vi "StimulationMode.vi"(8 "error in (no error)":errorcluster, 11 "SetupInfo_IN":T1={"ConfigParameters_Analog"={"JAI camera fps"=240.0, "Bi-Lateral Galvo xy scan range (V)"=0.7, "Bi-Lateral Galvo xy scan frequency (Hz)"=500, "AOM Blind percent (%)"=0.1, "AOM start blind percent (%) "=70.0, "ROI threshold"=1.0, "AO Sampling rate"=1000000.0}, "ConfigParameters_Digital"={"Steps per volume"=25.0, "Time per volume (s)"=0.4, "OG start layer"=15.0, "Objective Lin Rising Vel (micron/ms）"=1.0, "Image depth (micron)"=200.0, "OG latency (s)"=10.0, "OG repitation"=3.0, "OG end layer"=17.0, "Shock1 duration (s)"=0.001, "Shock2 duration (s)"=0.001, "Shock3 duration (s)"=0.01, "Shock4 duration (s)"=0.01, "Shock5 duration (s)"=0.1, "Shock duration_New"=[]}, "ConfigParameters_Other1"={"Frontal Galvo xy scan range (V)"=0.14, "Frontal Galvo xy scan frequency (Hz)"=500, "PFI 0 digital clock frequency"=500000.0, "Window size for layer index"=0.5, "sCMOS fps"=95.0}, "ConfigParameters_Others2"={"#Trials baseline"=6, "#Trials test"=6, "Time before acq. (s)"=360.0, "Time before test (s)"=600.0, "#Blocks acquisition"=5, "Inter-trial interval baseline (s)"=60.0, "#Trials per acquition block"=6, "Inter-block interval acquisition (s)"=360.0, "Inter-trial interval acquisition (s)"=20.0, "Flash latency (s)"=10.0, "Flash duration (s)"=3.2, "Response duration (s)"=10.0, "MaxTimeEventDetection (s)"=6, "StimType"=enum."Flash", "#MaxEvents"=6}, "ProcessParametersOut"={"stand Z vol Acquisition time (s)"=0.2631578947368421, "stand Z vol Backward time (s)"=0.13684210526315793, "Objective scan volt"=5.0, "Bi-lateral Galvo Z scan volt"=0.1800000180000018, "Frontal Galvo Z scan volt"=0.14940000509752818, "Objective step length (micron)"=8.0, "OG Z volet Linear Dec time (s)"=0.024, "OG Z vol Stim. steps time (s)"=0.031578947368421054, "OG Z vol Linear Acc time (s)"=0.112, "#Vol. of flash"=8, "#Vol. of shock"=1, "#Vol. bef flash"=25, "#Vol. aft flash"=17, "OG Z vol Linear Dec time (s)"=0.112, "OG Z vol time (s)"=0.39073684210526316, "Stack duration"=[0.001, 0.001, 0.01, 0.01, 0.1], "AOM stand. value size"=400000, "Plane indexing length"=0, "#Vol. blank"=0, "#Vol. blank before acq"=1000000, "#Vol. blank before test"=263158, " #Inter-block interval acquisition (Ed-St Vol)"=1000000}, "WaveformParameters"={"stand Z vol Acquisition samp info"={"Fs"=1000000.0, "#s"=263158.0}, "stand Z vol Backward samp info"={"Fs"=1000000.0, "#s"=136842.0}, "OG Z vol Linear Acc samp info"={"Fs"=1000000.0, "#s"=112000.0}, "OG Z vol Stim. steps samp info"={"Fs"=1000000.0, "#s"=31579.0}, "OG Z volet Linear Dec samp info"={"Fs"=1000000.0, "#s"=24000.0}, "OG Z vol Linear Dec samp info"={"Fs"=1000000.0, "#s"=112000.0}, "OG Z vol samp info"={"Fs"=1000000.0, "#s"=390737.0}, "stand Z vol backforth samp info"={"Fs"=1000000.0, "#s"=400000.0}}, "AnalogWaveform"={"Bi-lateral Galvo Z stand waveform"={"t0"=timestamp(0 s since 1904-01-01), "dt"=1.0, "Y"=[]}, "Frontal Galvo Z stand waveform"={"t0"=timestamp(0 s since 1904-01-01), "dt"=1.0, "Y"=[]}, "Bi-lateral Galvo XY stand waveform"={"t0"=timestamp(0 s since 1904-01-01), "dt"=1.0, "Y"=[]}, "Frontal Galvo XY stand waveform"={"t0"=timestamp(0 s since 1904-01-01), "dt"=1.0, "Y"=[]}, "sCMOS stand waveform"={"t0"=timestamp(0 s since 1904-01-01), "dt"=1.0, "Y"=[]}, "Detection objective stand waveform"={"t0"=timestamp(0 s since 1904-01-01), "dt"=1.0, "Y"=[]}, "AOM stand waveform"={"t0"=timestamp(0 s since 1904-01-01), "dt"=1.0, "Y"=[]}, "PFI 0 clock stand waveform"={"t0"=timestamp(0 s since 1904-01-01), "dt"=1.0, "Y"=[]}, "Bi-lateral Galvo Z OG waveform"={"t0"=timestamp(0 s since 1904-01-01), "dt"=1.0, "Y"=[]}, "Bi-lateral Galvo XY OG waveform"={"t0"=timestamp(0 s since 1904-01-01), "dt"=1.0, "Y"=[]}, "Frontal Galvo Z OG waveform"={"t0"=timestamp(0 s since 1904-01-01), "dt"=1.0, "Y"=[]}, "Frontal Galvo XY OG waveform"={"t0"=timestamp(0 s since 1904-01-01), "dt"=1.0, "Y"=[]}, "sCMOS OG waveform"={"t0"=timestamp(0 s since 1904-01-01), "dt"=1.0, "Y"=[]}, "Detection objective OG waveform"={"t0"=timestamp(0 s since 1904-01-01), "dt"=1.0, "Y"=[]}, "AOM OG waveform"={"t0"=timestamp(0 s since 1904-01-01), "dt"=1.0, "Y"=[]}, "PFI 0 clock OG wavee"={"t0"=timestamp(0 s since 1904-01-01), "dt"=1.0, "Y"=[]}, "sCMOS blank waveform"={"t0"=timestamp(0 s since 1904-01-01), "dt"=1.0, "Y"=[]}, "All analog OG wave"=[], "All analog stand wave"=[], "All analog blank wave"=[], "BufferWaveform_Analog"=[], "Bi-lateral Galvo Z XY"={"t0"=timestamp(0 s since 1904-01-01), "dt"=1.0, "Y"=[]}, "Frontal Galvo Z XY"={"t0"=timestamp(0 s since 1904-01-01), "dt"=1.0, "Y"=[]}, "sCMOS Trigger XY"={"t0"=timestamp(0 s since 1904-01-01), "dt"=1.0, "Y"=[]}, "Detection objective XY"={"t0"=timestamp(0 s since 1904-01-01), "dt"=1.0, "Y"=[]}, "AOM XY"={"t0"=timestamp(0 s since 1904-01-01), "dt"=1.0, "Y"=[]}, "Analog_XY"=[]}, "DigitalWaveform"={"AllDigitalStandWave"=[], "AllDigialEvokedWave"=[], "AllDigialOGWave"=[], "AllDigitalPairWave_1"=[], "AllDigitalPairWave_2"=[], "AllDigitalPairWave_3"=[], "AllDigitalPairWave_4"=[], "AllDigitalPairWave_5"=[], "Plane Indexing"={"t0"=timestamp(0 s since 1904-01-01), "dt"=0.0, "Y"={"transitions"=[], "data"=[]}, "error"={"status"=FALSE, "code"=37421928, "source"=""}}, "Plane indexing P0.5 OG"={"t0"=timestamp(0 s since 1904-01-01), "dt"=0.0, "Y"={"transitions"=[], "data"=[]}, "error"={"status"=FALSE, "code"=37421928, "source"=""}}, "AllDigitalPairWaves"=[], "BufferWaveform_Digital"=[], "AllDigitalBlankWave"=[], "Digial_XY"=[], "Digital_XY_flash"=[], "Digial_XY DMD"=[]}, "PhysicalResource"={"PhysicalChannels_AI"="", "PhysicalChannels_AO"="", "PhysicalChannels_DO"="", "Task_AnalogOutput"="", "Task_DigitalOutput"="", "Task_AnalogInput"=""}, "ControlsRef"={"Mode_1"=refnum, "EventDetectionMode"=refnum, "Mode_2A"=refnum, "StimulationMode"=refnum, "Mode_2B"=refnum, "ErrorMeg"=refnum}, "test"=""} {"ConfigParameters_Other1"."Frontal Galvo xy scan frequency (Hz)" min=500 max=500; "ConfigParameters_Other1"."Frontal Galvo xy scan range (V)" min=0.0 max=1.5; "ConfigParameters_Analog"."AOM start blind percent (%)" min=10.0 max=90.0; "ConfigParameters_Analog"."AOM Blind percent (%)" min=0.1 max=100.0; "ConfigParameters_Analog"."Bi-Lateral Galvo xy scan frequency (Hz)" min=500 max=500; "ConfigParameters_Analog"."Bi-Lateral Galvo xy scan range (V)" min=0.0 max=1.5}) -> (0 "error out":errorcluster, 3 "SetupInfo_OUT":T1={"ConfigParameters_Analog"={"JAI camera fps"=240.0, "Bi-Lateral Galvo xy scan range (V)"=0.7, "Bi-Lateral Galvo xy scan frequency (Hz)"=500, "AOM Blind percent (%)"=0.1, "AOM start blind percent (%) "=70.0, "ROI threshold"=1.0, "AO Sampling rate"=1000000.0}, "ConfigParameters_Digital"={"Steps per volume"=25.0, "Time per volume (s)"=0.4, "OG start layer"=15.0, "Objective Lin Rising Vel (micron/ms）"=1.0, "Image depth (micron)"=200.0, "OG latency (s)"=10.0, "OG repitation"=3.0, "OG end layer"=17.0, "Shock1 duration (s)"=0.001, "Shock2 duration (s)"=0.001, "Shock3 duration (s)"=0.01, "Shock4 duration (s)"=0.01, "Shock5 duration (s)"=0.1, "Shock duration_New"=[]}, "ConfigParameters_Other1"={"Frontal Galvo xy scan range (V)"=0.14, "Frontal Galvo xy scan frequency (Hz)"=500, "PFI 0 digital clock frequency"=500000.0, "Window size for layer index"=0.5, "sCMOS fps"=95.0}, "ConfigParameters_Others2"={"#Trials baseline"=6, "#Trials test"=6, "Time before acq. (s)"=360.0, "Time before test (s)"=600.0, "#Blocks acquisition"=5, "Inter-trial interval baseline (s)"=60.0, "#Trials per acquition block"=6, "Inter-block interval acquisition (s)"=360.0, "Inter-trial interval acquisition (s)"=20.0, "Flash latency (s)"=10.0, "Flash duration (s)"=3.2, "Response duration (s)"=10.0, "MaxTimeEventDetection (s)"=6, "StimType"=enum."Flash", "#MaxEvents"=6}, "ProcessParametersOut"={"stand Z vol Acquisition time (s)"=0.2631578947368421, "stand Z vol Backward time (s)"=0.13684210526315793, "Objective scan volt"=5.0, "Bi-lateral Galvo Z scan volt"=0.1800000180000018, "Frontal Galvo Z scan volt"=0.14940000509752818, "Objective step length (micron)"=8.0, "OG Z volet Linear Dec time (s)"=0.024, "OG Z vol Stim. steps time (s)"=0.031578947368421054, "OG Z vol Linear Acc time (s)"=0.112, "#Vol. of flash"=8, "#Vol. of shock"=1, "#Vol. bef flash"=25, "#Vol. aft flash"=17, "OG Z vol Linear Dec time (s)"=0.112, "OG Z vol time (s)"=0.39073684210526316, "Stack duration"=[0.001, 0.001, 0.01, 0.01, 0.1], "AOM stand. value size"=400000, "Plane indexing length"=0, "#Vol. blank"=0, "#Vol. blank before acq"=1000000, "#Vol. blank before test"=263158, " #Inter-block interval acquisition (Ed-St Vol)"=1000000}, "WaveformParameters"={"stand Z vol Acquisition samp info"={"Fs"=1000000.0, "#s"=263158.0}, "stand Z vol Backward samp info"={"Fs"=1000000.0, "#s"=136842.0}, "OG Z vol Linear Acc samp info"={"Fs"=1000000.0, "#s"=112000.0}, "OG Z vol Stim. steps samp info"={"Fs"=1000000.0, "#s"=31579.0}, "OG Z volet Linear Dec samp info"={"Fs"=1000000.0, "#s"=24000.0}, "OG Z vol Linear Dec samp info"={"Fs"=1000000.0, "#s"=112000.0}, "OG Z vol samp info"={"Fs"=1000000.0, "#s"=390737.0}, "stand Z vol backforth samp info"={"Fs"=1000000.0, "#s"=400000.0}}, "AnalogWaveform"={"Bi-lateral Galvo Z stand waveform"={"t0"=timestamp(0 s since 1904-01-01), "dt"=1.0, "Y"=[]}, "Frontal Galvo Z stand waveform"={"t0"=timestamp(0 s since 1904-01-01), "dt"=1.0, "Y"=[]}, "Bi-lateral Galvo XY stand waveform"={"t0"=timestamp(0 s since 1904-01-01), "dt"=1.0, "Y"=[]}, "Frontal Galvo XY stand waveform"={"t0"=timestamp(0 s since 1904-01-01), "dt"=1.0, "Y"=[]}, "sCMOS stand waveform"={"t0"=timestamp(0 s since 1904-01-01), "dt"=1.0, "Y"=[]}, "Detection objective stand waveform"={"t0"=timestamp(0 s since 1904-01-01), "dt"=1.0, "Y"=[]}, "AOM stand waveform"={"t0"=timestamp(0 s since 1904-01-01), "dt"=1.0, "Y"=[]}, "PFI 0 clock stand waveform"={"t0"=timestamp(0 s since 1904-01-01), "dt"=1.0, "Y"=[]}, "Bi-lateral Galvo Z OG waveform"={"t0"=timestamp(0 s since 1904-01-01), "dt"=1.0, "Y"=[]}, "Bi-lateral Galvo XY OG waveform"={"t0"=timestamp(0 s since 1904-01-01), "dt"=1.0, "Y"=[]}, "Frontal Galvo Z OG waveform"={"t0"=timestamp(0 s since 1904-01-01), "dt"=1.0, "Y"=[]}, "Frontal Galvo XY OG waveform"={"t0"=timestamp(0 s since 1904-01-01), "dt"=1.0, "Y"=[]}, "sCMOS OG waveform"={"t0"=timestamp(0 s since 1904-01-01), "dt"=1.0, "Y"=[]}, "Detection objective OG waveform"={"t0"=timestamp(0 s since 1904-01-01), "dt"=1.0, "Y"=[]}, "AOM OG waveform"={"t0"=timestamp(0 s since 1904-01-01), "dt"=1.0, "Y"=[]}, "PFI 0 clock OG wavee"={"t0"=timestamp(0 s since 1904-01-01), "dt"=1.0, "Y"=[]}, "sCMOS blank waveform"={"t0"=timestamp(0 s since 1904-01-01), "dt"=1.0, "Y"=[]}, "All analog OG wave"=[], "All analog stand wave"=[], "All analog blank wave"=[], "BufferWaveform_Analog"=[], "Bi-lateral Galvo Z XY"={"t0"=timestamp(0 s since 1904-01-01), "dt"=1.0, "Y"=[]}, "Frontal Galvo Z XY"={"t0"=timestamp(0 s since 1904-01-01), "dt"=1.0, "Y"=[]}, "sCMOS Trigger XY"={"t0"=timestamp(0 s since 1904-01-01), "dt"=1.0, "Y"=[]}, "Detection objective XY"={"t0"=timestamp(0 s since 1904-01-01), "dt"=1.0, "Y"=[]}, "AOM XY"={"t0"=timestamp(0 s since 1904-01-01), "dt"=1.0, "Y"=[]}, "Analog_XY"=[]}, "DigitalWaveform"={"AllDigitalStandWave"=[], "AllDigialEvokedWave"=[], "AllDigialOGWave"=[], "AllDigitalPairWave_1"=[], "AllDigitalPairWave_2"=[], "AllDigitalPairWave_3"=[], "AllDigitalPairWave_4"=[], "AllDigitalPairWave_5"=[], "Plane Indexing"={"t0"=timestamp(0 s since 1904-01-01), "dt"=0.0, "Y"={"transitions"=[], "data"=[]}, "error"={"status"=FALSE, "code"=37421928, "source"=""}}, "Plane indexing P0.5 OG"={"t0"=timestamp(0 s since 1904-01-01), "dt"=0.0, "Y"={"transitions"=[], "data"=[]}, "error"={"status"=FALSE, "code"=37421928, "source"=""}}, "AllDigitalPairWaves"=[], "BufferWaveform_Digital"=[], "AllDigitalBlankWave"=[], "Digial_XY"=[], "Digital_XY_flash"=[], "Digial_XY DMD"=[]}, "PhysicalResource"={"PhysicalChannels_AI"="", "PhysicalChannels_AO"="", "PhysicalChannels_DO"="", "Task_AnalogOutput"="", "Task_DigitalOutput"="", "Task_AnalogInput"=""}, "ControlsRef"={"Mode_1"=refnum, "EventDetectionMode"=refnum, "Mode_2A"=refnum, "StimulationMode"=refnum, "Mode_2B"=refnum, "ErrorMeg"=refnum}, "test"=""} {"ConfigParameters_Other1"."Frontal Galvo xy scan frequency (Hz)" min=500 max=500; "ConfigParameters_Other1"."Frontal Galvo xy scan range (V)" min=0.0 max=1.5; "ConfigParameters_Analog"."AOM start blind percent (%)" min=10.0 max=90.0; "ConfigParameters_Analog"."AOM Blind percent (%)" min=0.1 max=100.0; "ConfigParameters_Analog"."Bi-Lateral Galvo xy scan frequency (Hz)" min=500 max=500; "ConfigParameters_Analog"."Bi-Lateral Galvo xy scan range (V)" min=0.0 max=1.5})   [LabVIEW 2018]
uses:
  SetupInfo.ctl
  ConfigParameters_Analog.ctl
  ConfigParameters_Digital.ctl
  ConfigParameters_Others1.ctl
  ConfigParameters_Others2.ctl
  ProcessParametersOut.ctl
  WaveformParameters.ctl
  AnalogWaveform.ctl
  DigitalWaveform.ctl
  PhysicalResource.ctl
  ControlsRef.ctl
  <vilib>/DAQmx/write.llb/DAQmx Write (Analog DBL 1Chan 1Samp).vi
  <vilib>/Analysis/baseanly.llb/Mean (DBL).vi
  <vilib>/DAQmx/create/channels.llb/DAQmx Create Channel (AO-Voltage-Basic).vi
  <vilib>/DAQmx/miscellaneous.llb/DAQmx Fill In Error Info.vi
  Trigger_Global.vi
  <vilib>/Analysis/NI_AALBase.lvlib
panel:
  out "OG?":bool
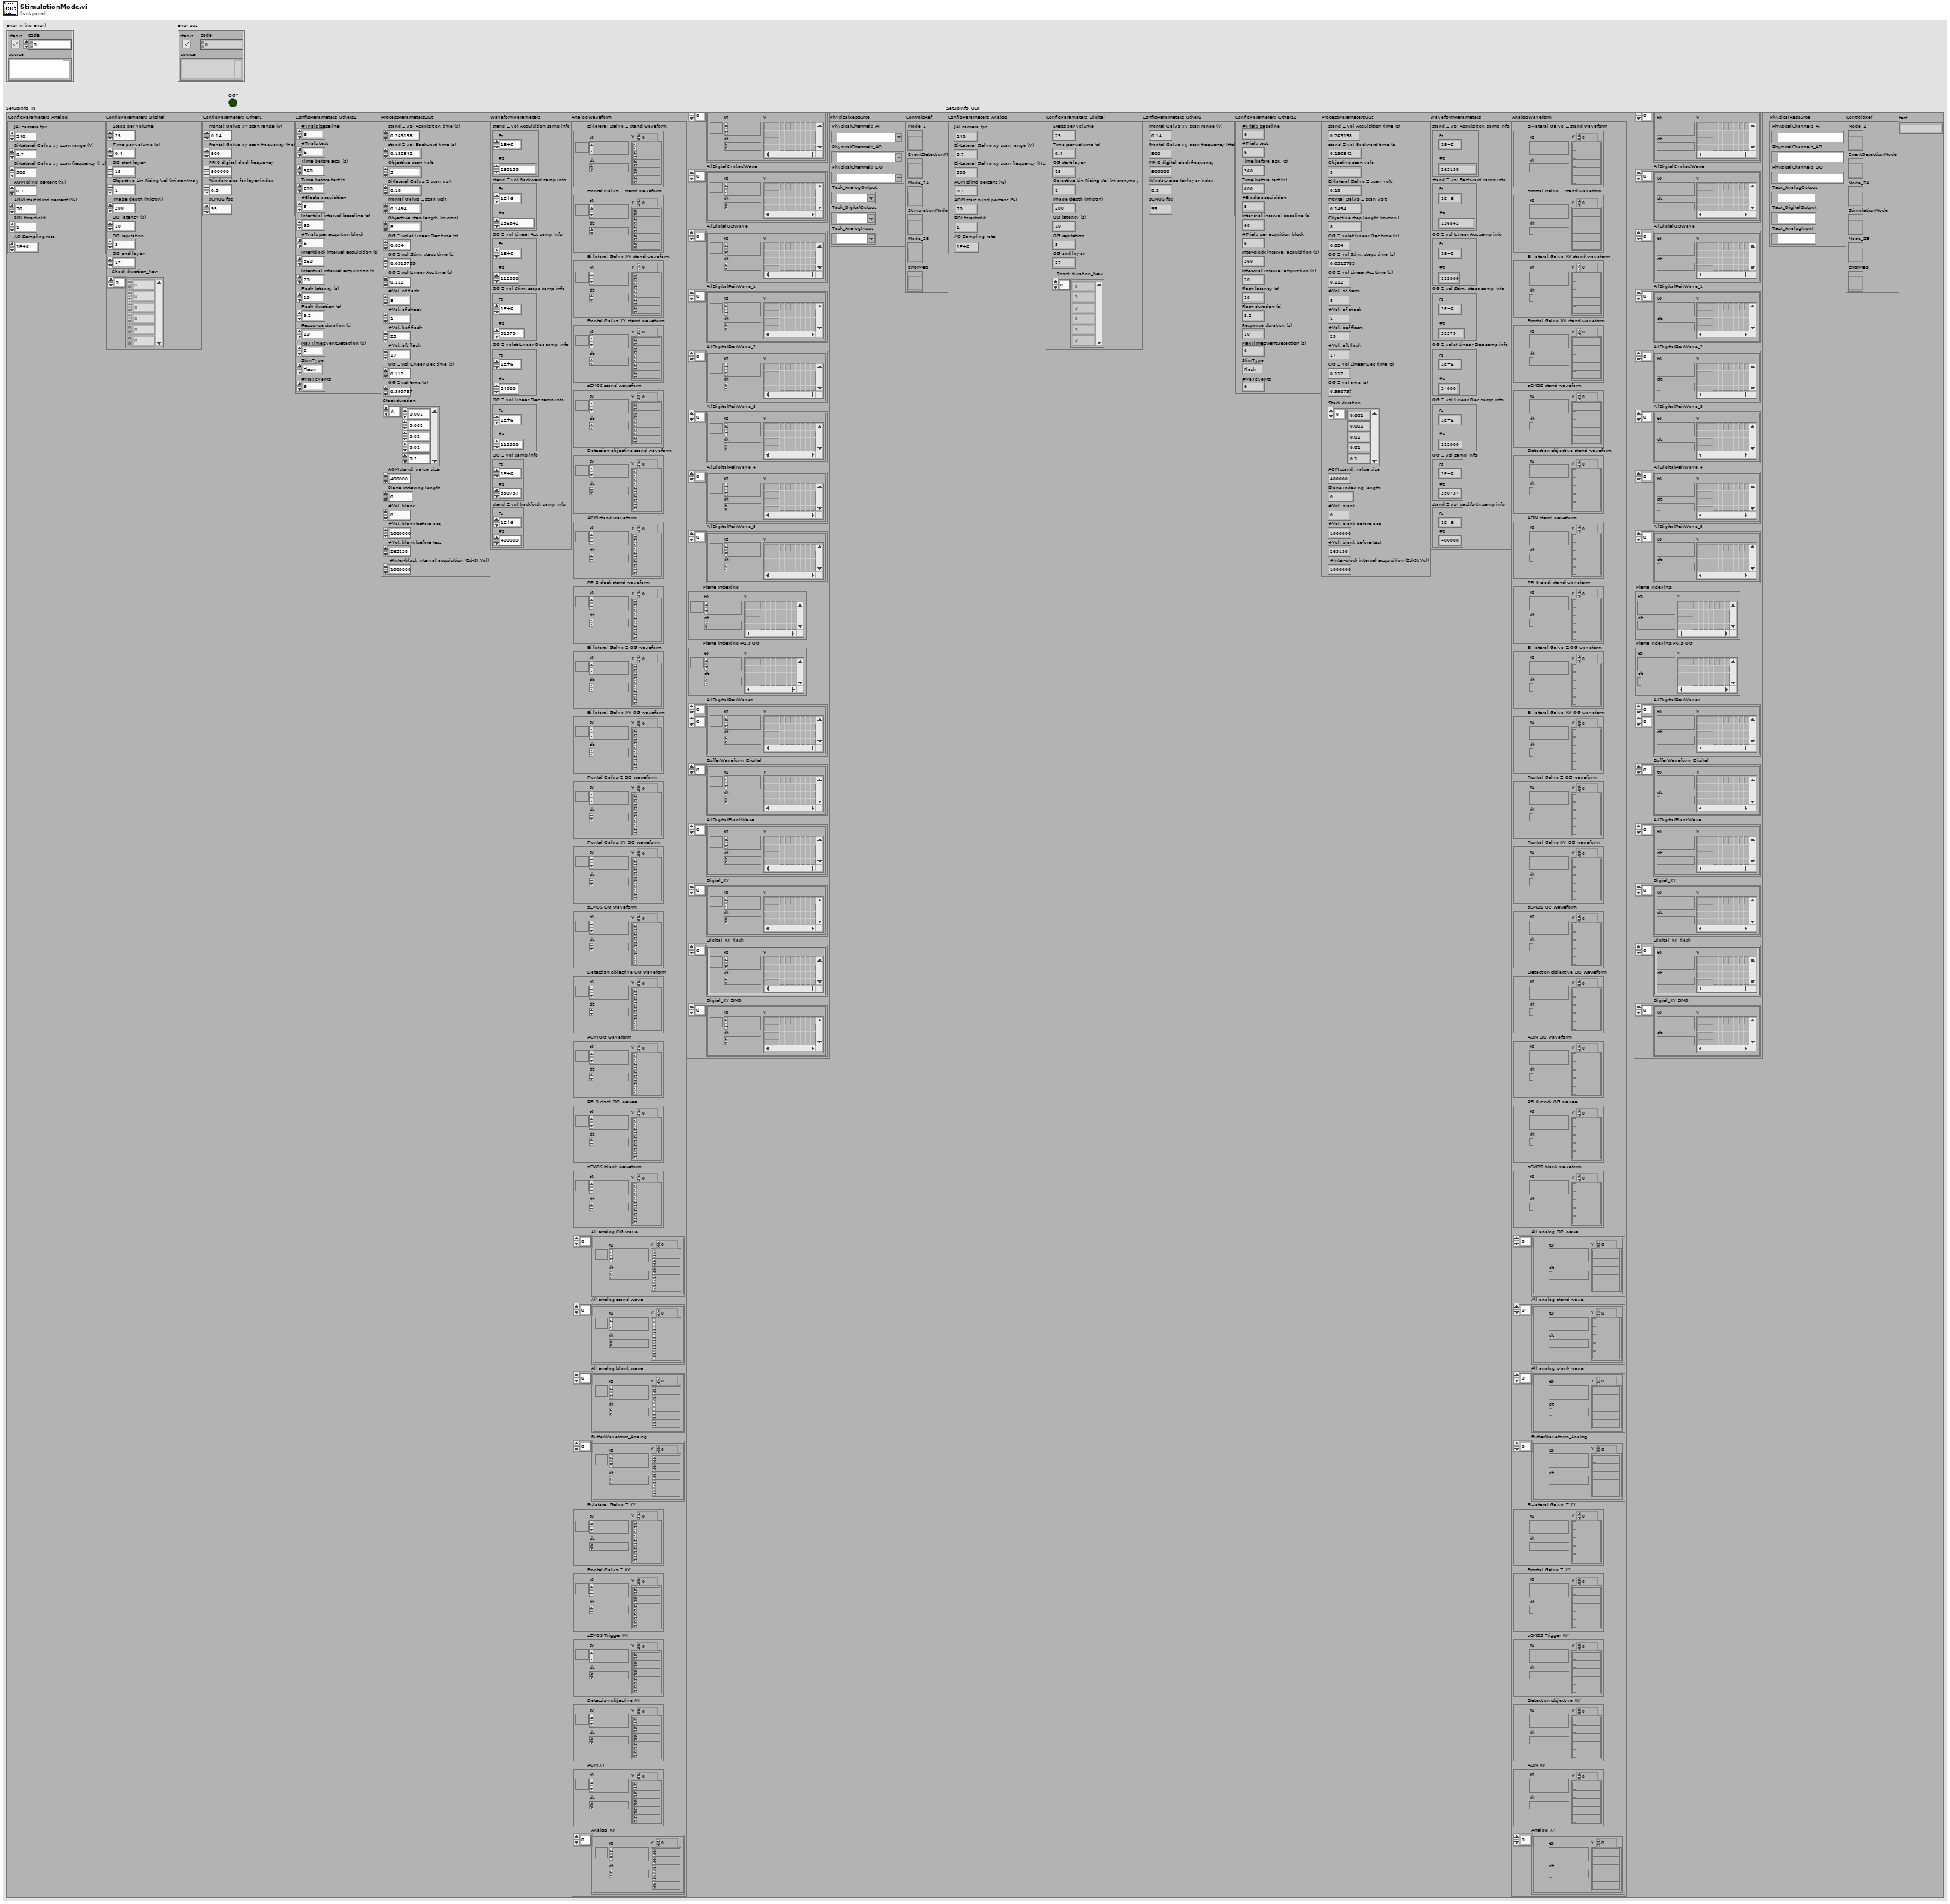
[diagram p1: front panel]
types:
  T1 = typedef "SetupInfo.ctl" = cluster{"ConfigParameters_Analog":T2, "ConfigParameters_Digital":T3, "ConfigParameters_Other1":T4, "ConfigParameters_Others2":T5, "ProcessParametersOut":T6, "WaveformParameters":T7, "AnalogWaveform":T8, "DigitalWaveform":T9, "PhysicalResource":T10, "ControlsRef":T11, "test":string}
  T2 = typedef "ConfigParameters_Analog.ctl" = cluster{"JAI camera fps":dbl, "Bi-Lateral Galvo xy scan range (V)":dbl, "Bi-Lateral Galvo xy scan frequency (Hz)":i16, "AOM Blind percent (%)":dbl, "AOM start blind percent (%) ":dbl, "ROI threshold":dbl, "AO Sampling rate":dbl}
  T3 = typedef "ConfigParameters_Digital.ctl" = cluster{"Steps per volume":dbl, "Time per volume (s)":dbl, "OG start layer":dbl, "Objective Lin Rising Vel (micron/ms）":dbl, "Image depth (micron)":dbl, "OG latency (s)":dbl, "OG repitation":dbl, "OG end layer":dbl, "Shock1 duration (s)":dbl, "Shock2 duration (s)":dbl, "Shock3 duration (s)":dbl, "Shock4 duration (s)":dbl, "Shock5 duration (s)":dbl, "Shock duration_New":dbl[]}
  T4 = typedef "ConfigParameters_Others1.ctl" = cluster{"Frontal Galvo xy scan range (V)":dbl, "Frontal Galvo xy scan frequency (Hz)":i16, "PFI 0 digital clock frequency":dbl, "Window size for layer index":dbl, "sCMOS fps":dbl}
  T5 = typedef "ConfigParameters_Others2.ctl" = cluster{"#Trials baseline":i32, "#Trials test":i32, "Time before acq. (s)":dbl, "Time before test (s)":dbl, "#Blocks acquisition":i32, "Inter-trial interval baseline (s)":dbl, "#Trials per acquition block":i32, "Inter-block interval acquisition (s)":dbl, "Inter-trial interval acquisition (s)":dbl, "Flash latency (s)":dbl, "Flash duration (s)":dbl, "Response duration (s)":dbl, "MaxTimeEventDetection (s)":i32, "StimType":enum16{"Flash", "OG"}, "#MaxEvents":i32}
  T6 = typedef "ProcessParametersOut.ctl" = cluster{"stand Z vol Acquisition time (s)":dbl, "stand Z vol Backward time (s)":dbl, "Objective scan volt":dbl, "Bi-lateral Galvo Z scan volt":dbl, "Frontal Galvo Z scan volt":dbl, "Objective step length (micron)":dbl, "OG Z volet Linear Dec time (s)":dbl, "OG Z vol Stim. steps time (s)":dbl, "OG Z vol Linear Acc time (s)":dbl, "#Vol. of flash":i32, "#Vol. of shock":i32, "#Vol. bef flash":i32, "#Vol. aft flash":i32, "OG Z vol Linear Dec time (s)":dbl, "OG Z vol time (s)":dbl, "Stack duration":dbl[], "AOM stand. value size":i32, "Plane indexing length":i32, "#Vol. blank":i32, "#Vol. blank before acq":i32, "#Vol. blank before test":i32, " #Inter-block interval acquisition (Ed-St Vol)":i32}
  T7 = typedef "WaveformParameters.ctl" = cluster{"stand Z vol Acquisition samp info":cluster{"Fs":dbl, "#s":dbl}, "stand Z vol Backward samp info":cluster{"Fs":dbl, "#s":dbl}, "OG Z vol Linear Acc samp info":cluster{"Fs":dbl, "#s":dbl}, "OG Z vol Stim. steps samp info":cluster{"Fs":dbl, "#s":dbl}, "OG Z volet Linear Dec samp info":cluster{"Fs":dbl, "#s":dbl}, "OG Z vol Linear Dec samp info":cluster{"Fs":dbl, "#s":dbl}, "OG Z vol samp info":cluster{"Fs":dbl, "#s":dbl}, "stand Z vol backforth samp info":cluster{"Fs":dbl, "#s":dbl}}
  T8 = typedef "AnalogWaveform.ctl" = cluster{"Bi-lateral Galvo Z stand waveform":waveform(dbl), "Frontal Galvo Z stand waveform":waveform(dbl), "Bi-lateral Galvo XY stand waveform":waveform(dbl), "Frontal Galvo XY stand waveform":waveform(dbl), "sCMOS stand waveform":waveform(dbl), "Detection objective stand waveform":waveform(dbl), "AOM stand waveform":waveform(dbl), "PFI 0 clock stand waveform":waveform(dbl), "Bi-lateral Galvo Z OG waveform":waveform(dbl), "Bi-lateral Galvo XY OG waveform":waveform(dbl), "Frontal Galvo Z OG waveform":waveform(dbl), "Frontal Galvo XY OG waveform":waveform(dbl), "sCMOS OG waveform":waveform(dbl), "Detection objective OG waveform":waveform(dbl), "AOM OG waveform":waveform(dbl), "PFI 0 clock OG wavee":waveform(dbl), "sCMOS blank waveform":waveform(dbl), "All analog OG wave":waveform(dbl)[], "All analog stand wave":waveform(dbl)[], "All analog blank wave":waveform(dbl)[], "BufferWaveform_Analog":waveform(dbl)[], "Bi-lateral Galvo Z XY":waveform(dbl), "Frontal Galvo Z XY":waveform(dbl), "sCMOS Trigger XY":waveform(dbl), "Detection objective XY":waveform(dbl), "AOM XY":waveform(dbl), "Analog_XY":waveform(dbl)[]}
  T9 = typedef "DigitalWaveform.ctl" = cluster{"AllDigitalStandWave":digitalwaveform[], "AllDigialEvokedWave":digitalwaveform[], "AllDigialOGWave":digitalwaveform[], "AllDigitalPairWave_1":digitalwaveform[], "AllDigitalPairWave_2":digitalwaveform[], "AllDigitalPairWave_3":digitalwaveform[], "AllDigitalPairWave_4":digitalwaveform[], "AllDigitalPairWave_5":digitalwaveform[], "Plane Indexing":digitalwaveform, "Plane indexing P0.5 OG":digitalwaveform, "AllDigitalPairWaves":digitalwaveform[][], "BufferWaveform_Digital":digitalwaveform[], "AllDigitalBlankWave":digitalwaveform[], "Digial_XY":digitalwaveform[], "Digital_XY_flash":digitalwaveform[], "Digial_XY DMD":digitalwaveform[]}
  T10 = typedef "PhysicalResource.ctl" = cluster{"PhysicalChannels_AI":tag, "PhysicalChannels_AO":tag, "PhysicalChannels_DO":tag, "Task_AnalogOutput":refnum<k21>, "Task_DigitalOutput":refnum<k21>, "Task_AnalogInput":refnum<k21>}
  T11 = typedef "ControlsRef.ctl" = cluster{"Mode_1":refnum<vi>, "EventDetectionMode":refnum<vi>, "Mode_2A":refnum<vi>, "StimulationMode":refnum<vi>, "Mode_2B":refnum<vi>, "ErrorMeg":refnum<vi>}
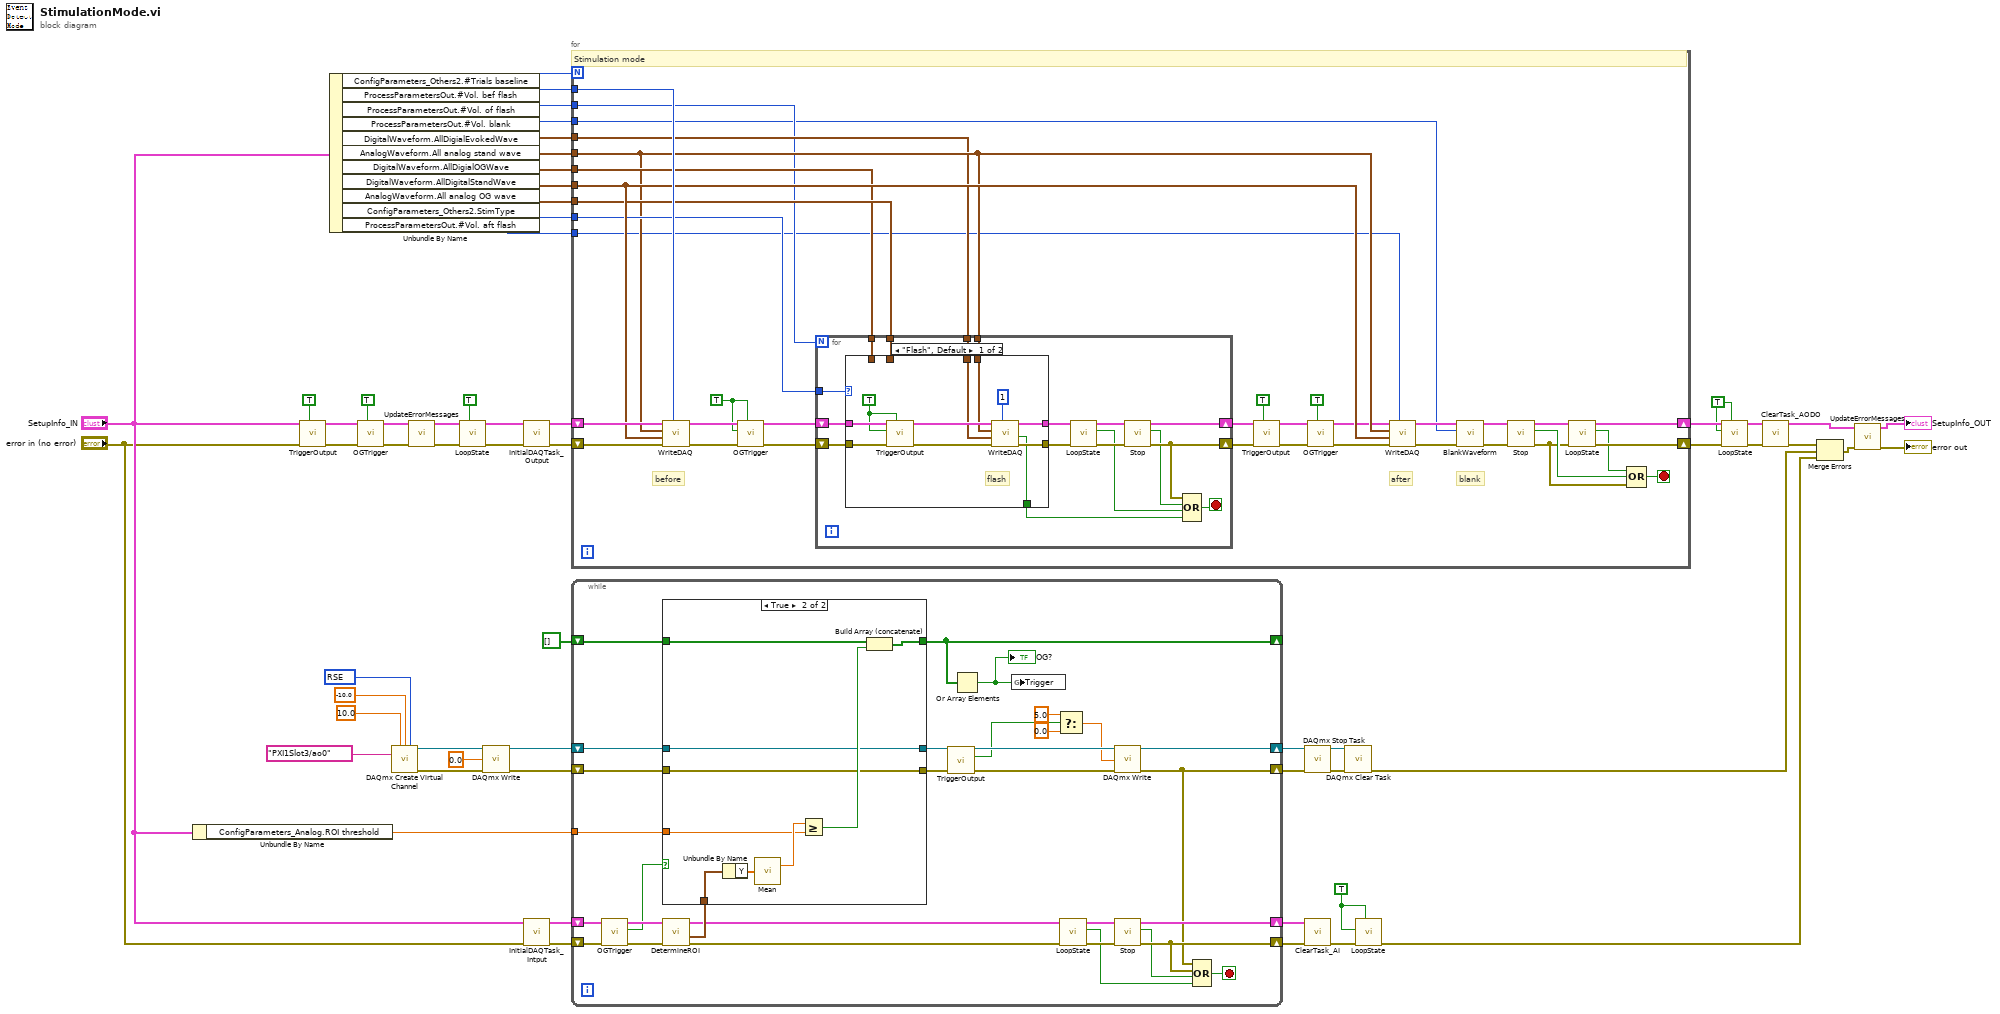
[diagram p0: block diagram]
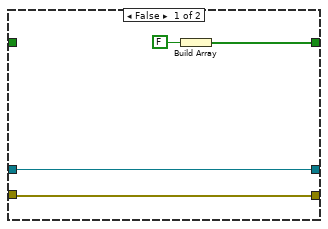
[diagram p2: hidden frame]
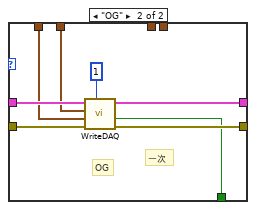
[diagram p3: hidden frame]
diagram:
  w16 = 10083 items=["Default"=-1, "RSE"=10083, "Differential"=10106, "Pseudodifferential"=12529] ("output terminal configuration")
  w23 = TRUE ("Write?")
  w40 = TRUE ("Write?")
  n1 = Unbundle By Name("SetupInfo_IN") -> ("ConfigParameters_Analog.ROI threshold"=w4:dbl)
  n2 = call "TriggerOutput.vi"("Write?"=TRUE, "error in (no error)"="error in (no error)") -> ("error out"=w2:errorcluster)  [unwired: 8 in, 1 out]
  n3 = Unbundle By Name("SetupInfo_IN") -> ("ConfigParameters_Others2.#Trials baseline"=w55:i32, "ProcessParametersOut.#Vol. bef flash"=w54:i32, "ProcessParametersOut.#Vol. of flash"=w53:i32, "ProcessParametersOut.#Vol. blank"=w52:i32, "DigitalWaveform.AllDigialEvokedWave"=w38:digitalwaveform[], "AnalogWaveform.All analog stand wave"=w51:waveform(dbl)[], "DigitalWaveform.AllDigialOGWave"=w50:digitalwaveform[], "DigitalWaveform.AllDigitalStandWave"=w49:digitalwaveform[], "AnalogWaveform.All analog OG wave"=w45:waveform(dbl)[], "ConfigParameters_Others2.StimType"=w39:enum16{"Flash", "OG"}, "ProcessParametersOut.#Vol. aft flash"=w37:i32)
  n4 = call "OGTrigger.vi"("Write?"=TRUE, "error in (no error)"=w2) -> ("error out"=w29:errorcluster)  [unwired: 8 in, 1 out]
  n5 = call-poly <vilib>:"DAQmx Create Virtual Channel.vi"("maximum value"=10.0, "minimum value"=-10.0, "output terminal configuration"=w16, "physical channels"=tag "PXI1Slot3/ao0") -> ("task out"=w12:refnum<k21>, "error out"=w11:errorcluster)  [unwired: 10 in]
  n6 = call "UpdateErrorMessages.vi"("error in (no error)"=w29, "SetupInfo_IN"="SetupInfo_IN") -> ("error out"=w30:errorcluster, "SetupInfo_OUT"=w31:T1)  [unwired: 8 in]
  n7 = call "LoopState.vi"("Write?"=TRUE, "error in (no error)"=w30) -> ("error out"=w36:errorcluster)  [unwired: 8 in, 1 out]
  n8 = call-poly <vilib>:"DAQmx Write.vi"("task/channels in"=w12, "data"=0.0, "error in"=w11) -> ("task out"=w9:refnum<k21>, "error out"=w10:errorcluster)  [unwired: 10 in, 1 out]
  n9 = call "InitialDAQTask_Output.vi"("error in (no error)"=w36, "SetupInfo_IN"=w31) -> ("error out"=w47:errorcluster, "SetupInfo_OUT"=w48:T1)  [unwired: 8 in]
  n10 = call "InitialDAQTask_Intput.vi"("error in (no error)"="error in (no error)", "SetupInfo_IN"="SetupInfo_IN") -> ("error out"=w27:errorcluster, "SetupInfo_OUT"=w24:T1)  [unwired: 8 in]
  n11 = for {
    N: w55 -> [_]
    shift-right: [w71] -> w41
    shift-left: w47 -> [w85]
    tunnel: w54 -> [w83]
    shift-right: [w69] -> w46
    shift-left: w48 -> [w84]
    tunnel: w53 -> [w75]
    tunnel: w52 -> [w65]
    tunnel: w51 -> [w77]
    tunnel: w50 -> [w78]
    tunnel: w49 -> [w82]
    tunnel: w45 -> [w79]
    tunnel: w39 -> [w81]
    tunnel: w38 -> [w76]
    tunnel: w37 -> [w74]
    stop <- w86 stop-if-true
    w62 = TRUE ("Write?")
    # "after"
    # "blank"
    # "before"
    # "Stimulation mode"
    n12 = call "WriteDAQ.vi"("Cycle"=w83, "error in (no error)"=w85, "DigitalWaveform_In"=w82, "AnalogWaveform_In"=w77, "SetupInfo_IN"=w84) -> ("error out"=w63:errorcluster, "SetupInfo_OUT"=w80:T1)  [unwired: 4 in, 1 out]
    n13 = call "OGTrigger.vi"("Write?"=w62, "error in (no error)"=w63, "StateIn"=w62) -> ("error out"=w64:errorcluster)  [unwired: 7 in, 1 out]
    n14 = for {
      N: w75 -> [_]
      tunnel: w81 -> [w100]
      tunnel: w79 -> [w97]
      tunnel: w78 -> [w96]
      tunnel: w77 -> [w95]
      tunnel: w76 -> [w94]
      shift-right: [w93] -> w56
      shift-left: w64 -> [w101]
      shift-right: [w98] -> w61
      shift-left: w80 -> [w99]
      stop <- w91 stop-if-true
      n15 = case shown="\"Flash\", Default" w100 {
        tunnel: w101 -> [w105 w119]
        tunnel: w99 -> [w109 w118]
        tunnel: [w110 w117] -> w98
        tunnel: [w111 w116] -> w90
        tunnel: w97 -> [_ w114]
        tunnel: w96 -> [_ w113]
        tunnel: w95 -> [w107 _]
        tunnel: w94 -> [w106 _]
        tunnel: [w102 w112] -> w87
        frame "Flash", Default {
          w103 = TRUE ("Write?")
          # "flash"
          n16 = call "TriggerOutput.vi"("Write?"=w103, "error in (no error)"=w105, "StateIn"=w103) -> ("error out"=w104:errorcluster)  [unwired: 7 in, 1 out]
          n17 = call "WriteDAQ.vi"("Cycle"=1, "error in (no error)"=w104, "DigitalWaveform_In"=w106, "AnalogWaveform_In"=w107, "SetupInfo_IN"=w109) -> ("error out"=w111:errorcluster, "Trigger"=w102:bool, "SetupInfo_OUT"=w110:T1)  [unwired: 4 in]
        }
        frame "OG" {
          # "一次"
          # "OG"
          n18 = call "WriteDAQ.vi"("Cycle"=1, "error in (no error)"=w119, "DigitalWaveform_In"=w113, "AnalogWaveform_In"=w114, "SetupInfo_IN"=w118) -> ("error out"=w116:errorcluster, "Trigger"=w112:bool, "SetupInfo_OUT"=w117:T1)  [unwired: 4 in]
        }
      }
      n19 = call "LoopState.vi"("error in (no error)"=w90) -> ("error out"=w89:errorcluster, "StateOut"=w88:bool)  [unwired: 9 in]
      n20 = call "Stop.vi"("error in (no error)"=w89) -> ("error out"=w93:errorcluster, "StateOut"=w92:bool)  [unwired: 9 in]
      n21 = Compound Arithmetic op=OR(w93, w92, w88, w87) -> (w91:bool)
    }
    n22 = call "TriggerOutput.vi"("Write?"=TRUE, "error in (no error)"=w56) -> ("error out"=w57:errorcluster)  [unwired: 8 in, 1 out]
    n23 = call "OGTrigger.vi"("Write?"=TRUE, "error in (no error)"=w57) -> ("error out"=w60:errorcluster)  [unwired: 8 in, 1 out]
    n24 = call "WriteDAQ.vi"("Cycle"=w74, "error in (no error)"=w60, "DigitalWaveform_In"=w82, "AnalogWaveform_In"=w77, "SetupInfo_IN"=w61) -> ("error out"=w67:errorcluster, "SetupInfo_OUT"=w66:T1)  [unwired: 4 in, 1 out]
    n25 = call "BlankWaveform.vi"("error in (no error)"=w67, "Cycle"=w65, "SetupInfo_IN"=w66) -> ("error out"=w68:errorcluster, "SetupInfo_OUT"=w69:T1)  [unwired: 7 in]
    n26 = call "Stop.vi"("error in (no error)"=w68) -> ("error out"=w72:errorcluster, "StateOut"=w73:bool)  [unwired: 9 in]
    n27 = call "LoopState.vi"("error in (no error)"=w72) -> ("error out"=w71:errorcluster, "StateOut"=w70:bool)  [unwired: 9 in]
    n28 = Compound Arithmetic op=OR(w70, w73, w72) -> (w86:bool)
  }
  n29 = while {
    shift-right: [w146] -> w26
    shift-left: w27 -> [w138]
    shift-right: [w140] -> w25
    shift-left: w24 -> [w136]
    shift-right: [w134] -> _
    shift-left: bool[] [] -> [w135]
    shift-right: [w129] -> w13
    shift-left: w9 -> [w132]
    shift-right: [w123] -> w14
    shift-left: w10 -> [w130]
    tunnel: w4 -> [w121]
    stop <- w144 stop-if-true
    n30 = call "OGTrigger.vi"("error in (no error)"=w138) -> ("error out"=w139:errorcluster, "StateOut"=w133:bool)  [unwired: 9 in]
    n31 = call "DetermineROI.vi"("error in (no error)"=w139, "SetupInfo_IN"=w136) -> ("error out"=w137:errorcluster, "data"=w141:waveform(dbl), "SetupInfo_OUT"=w140:T1)  [unwired: 7 in]
    n32 = case shown="True" w133 {
      tunnel: w141 -> [_ w154]
      tunnel: [w149 w155] -> w134
      tunnel: w135 -> [_ w157]
      tunnel: w132 -> [w148 w153]
      tunnel: [w148 w153] -> w131
      tunnel: [w147 w152] -> w128
      tunnel: w130 -> [w147 w152]
      tunnel: w121 -> [_ w151]
      frame False {
        n33 = Build Array(FALSE) -> (w149:bool[])
      }
      frame True {
        n34 = Unbundle By Name(w154) -> ("Y"=w158:dbl[])
        n35 = call-poly <vilib>:"Mean.vi"("X"=w158) -> ("mean"=w159:dbl)  [unwired: 1 out]
        n36 = Greater Or Equal?(x=w159, y=w151) -> (x >= y?=w156:bool)
        n37 = Build Array (concatenate)(w157, w156) -> (w155:bool[])
      }
    }
    n38 = call "TriggerOutput.vi"("error in (no error)"=w128) -> ("error out"=w127:errorcluster, "StateOut"=w120:bool)  [unwired: 9 in]
    n39 = Or Array Elements(Boolean array=w134) -> (logical OR=w122:bool)
    "OG?" <- w122
    n40 = global write "Trigger_Global.vi" "Trigger"(w122) -> ()
    n41 = Select(t=5.0, s=w120, f=0.0 ("data")) -> (s? t:f=w124:dbl)
    n42 = call "LoopState.vi"("error in (no error)"=w137) -> ("error out"=w143:errorcluster, "StateOut"=w142:bool)  [unwired: 9 in]
    n43 = call-poly <vilib>:"DAQmx Write.vi"("task/channels in"=w131, "data"=w124, "error in"=w127) -> ("task out"=w129:refnum<k21>, "error out"=w123:errorcluster)  [unwired: 10 in, 1 out]
    n44 = call "Stop.vi"("error in (no error)"=w143) -> ("error out"=w146:errorcluster, "StateOut"=w145:bool)  [unwired: 9 in]
    n45 = Compound Arithmetic op=OR(w123, w146, w145, w142) -> (w144:bool)
  }
  n46 = call <vilib>:"DAQmx Stop Task.vi"("task/channels in"=w13, "error in"=w14) -> ("task out"=w20:refnum<k21>, "error out"=w19:errorcluster)  [unwired: 12 in]
  n47 = call "ClearTask_AI.vi"("error in (no error)"=w26, "SetupInfo_IN"=w25) -> ("error out"=w22:errorcluster)  [unwired: 8 in, 1 out]
  n48 = call <vilib>:"DAQmx Clear Task.vi"("task in"=w20, "error in"=w19) -> ("error out"=w6:errorcluster)  [unwired: 13 in]
  n49 = call "LoopState.vi"("Write?"=w23, "error in (no error)"=w22, "StateIn"=w23) -> ("error out"=w7:errorcluster)  [unwired: 7 in, 1 out]
  n50 = call "LoopState.vi"("Write?"=w40, "error in (no error)"=w41, "StateIn"=w40) -> ("error out"=w42:errorcluster)  [unwired: 7 in, 1 out]
  n51 = call "ClearTask_AODO.vi"("error in (no error)"=w42, "SetupInfo_IN"=w46) -> ("error out"=w44:errorcluster, "SetupInfo_OUT"=w33:T1)  [unwired: 8 in]
  n52 = Merge Errors(w44, w6, w7) -> (w35:errorcluster)
  n53 = call "UpdateErrorMessages.vi"("error in (no error)"=w35, "SetupInfo_IN"=w33) -> ("error out"=→"error out":errorcluster, "SetupInfo_OUT"=→"SetupInfo_OUT":T1)  [unwired: 8 in]
